vi "set array to last element.vi"(0 "Arr Refnum":refnum<vi>) -> ()   [LabVIEW 2018]
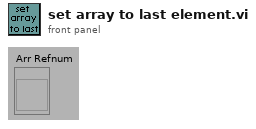
[diagram p1: front panel]
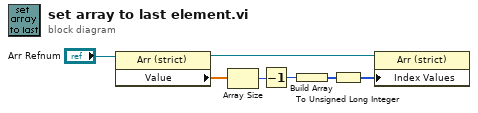
[diagram p0: block diagram]
diagram:
  n1 = property class="Arr (strict)"(reference="Arr Refnum") -> (reference out=w2:refnum<vi>, "Value"=w6:dbl[])  [unwired: 1 in, 1 out]
  n2 = Array Size(array=w6) -> (size(s)=w4:i32)
  n3 = Decrement(x=w4) -> (x-1=w5:i32)
  n4 = Build Array(w5) -> (w3:i32[])
  n5 = To Unsigned Long Integer(number=w3) -> (unsigned 32bit integer=w1:u32[])
  n6 = property class="Arr (strict)"(reference=w2, "Index Values"=w1) -> ()  [unwired: 1 in, 2 out]
